vi "UI Front Panel State.vi"(8 "error in (no error)":errorcluster, 9 "Front Panel Window:Behavior":T1(ring)=enum."Default", 10 "Argument":T2="Open", 11 "UI ActorTop in":refnum<class "UI_Top_Customer.lvclass">) -> (0 "error out":errorcluster, 3 "UI ActorTop out":refnum<class "UI_Top_Customer.lvclass">)   [LabVIEW 2021, in "UI_Top_Customer.lvclass"]
doc: "UI: Front Panel State\ninclude Open, close, standard, Hidden and FP.Center\n2015-03-18 16:41:03\n蒋松\njiangsong@outlook.com"
uses:
  UI_Top_Customer.lvclass
  <userlib>/John_Lib/Control/Panel State.ctl
  UI_Top_Customer.lvclass/UI_Top_Customer.ctl
  <userlib>/John_Lib/AbstractActorTemplate/AbstractActorTemplate/UIActorTop.lvclass
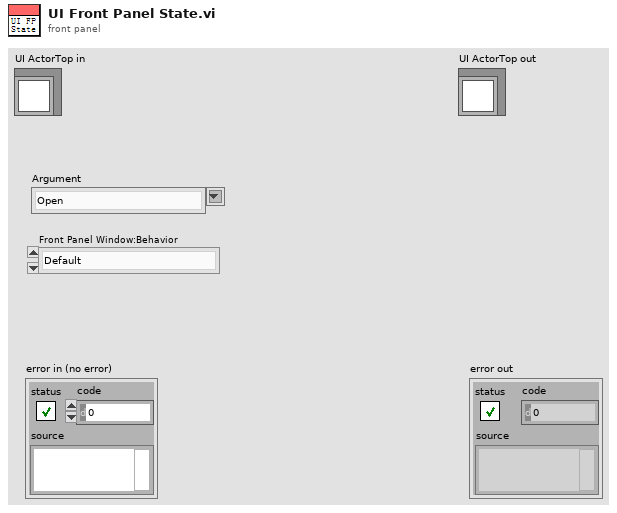
[diagram p1: front panel]
types:
  T1 = enum32{"Invalid", "Default", "Floating", "Floating/Auto-Hide", "Modal"}
  T2 = typedef "Panel State.ctl" = string
  T3 = typedef "UI_Top_Customer.lvlib/UI_Top_Customer.lvclass/Pane MouseDown.ctl" = cluster{"Type":T4, "Coords":T5, "Mods":cluster{"Double Click":bool, "Menu Key":bool}, "Pane: MouseDown":bool}
  T4 = typedef "lveventtype.ctl" = enum32{"Null", "Timeout", "Annotation Menu Selection", "Annotation Menu Selection?", "App Instance Close", "App Instance Close?", "Autoscale Range Change", "Bookmark Info Change", "Cell Edit", "Cell Edit?", "Cursor Grab", "Cursor Grab?", "Cursor Menu Selection", "Cursor Menu Selection?", "Cursor Move", "Cursor Release", "Data Change", "Direction Change", "Display State Change", "Drag Ended", "Drag Enter", "Drag Leave", "Drag Over", "Drag Source Update", "Drag Starting", "Drag Starting?", "Drop", "Exec State Change", "Key Down", "Key Down?", "Key Repeat", "Key Repeat?", "Key Up", "Listbox Double Click", "Menu Activation?", "Menu Selection (App)", "Menu Selection? (App)", "Menu Selection (User)", "Mouse Down", "Mouse Down?", "Mouse Enter", "Mouse Leave", "Mouse Move", "Mouse Up", "Mouse Wheel", "NI Security User Change (App)", "Pane Size", "Panel Close", "Panel Close?", "Panel Resize", "Plot Attribute Change", "Scale Range Change", "Shortcut Menu Activation?", "Shortcut Menu Selection (App)", "Shortcut Menu Selection? (App)", "Shortcut Menu Selection (User)", "Tree Double Click", "Tree Drag", "Tree Drag?", "Tree Drop", "Tree Drop?", "Tree Item Close", "Tree Item Close?", "Tree Item Open", "Tree Item Open?", "User Event", "Value Change"}
  T5 = typedef "LVPoint32TypeDef.ctl" = cluster{"Horizontal":i32, "Vertical":i32}
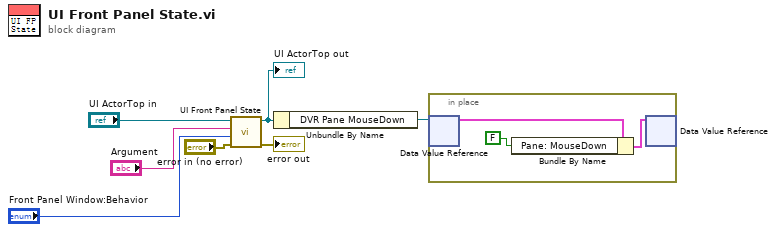
[diagram p0: block diagram]
diagram:
  n1 = call-parent "UI Front Panel State.vi"("error in (no error)"="error in (no error)", "Front Panel Window:Behavior"="Front Panel Window:Behavior", "Argument"="Argument", "UI ActorTop in"="UI ActorTop in") -> ("error out"=→"error out":errorcluster, "UI ActorTop out"=w1:refnum<class "UI_Top_Customer.lvclass">)  [unwired: 6 in]
  "UI ActorTop out" <- w1
  n2 = Unbundle By Name(w1) -> ("DVR Pane MouseDown"=w2:refnum<data-value>)
  n3 = in-place {
    n4 = in-place-dvr #1(w2) -> (w10:T3)  [unwired: 1 out]
    n5 = Bundle By Name(cluster=w10, "Pane: MouseDown"=FALSE) -> (w9:T3)
    n6 = in-place-dvr #1(w9) -> ()  [unwired: 2 out]
  }
